vi "query_vectorsearch.vi"(0 "abstract_vector_base in":refnum<class "abstract_vector_base.lvclass">, 5 "collection_name":string, 7 "vector":dbl[](array[numeric]), 9 "limit":u32, 11 "error in (no error)":errorcluster) -> (4 "abstract_vector_base out":refnum<class "abstract_vector_base.lvclass">, 6 "results":T1[](array[typedef]), 15 "error out":errorcluster)   [LabVIEW 2020, in "abstract_vector_base.lvclass"]
uses:
  abstract_vector_base.lvclass
  search result.ctl
  vector.ctl
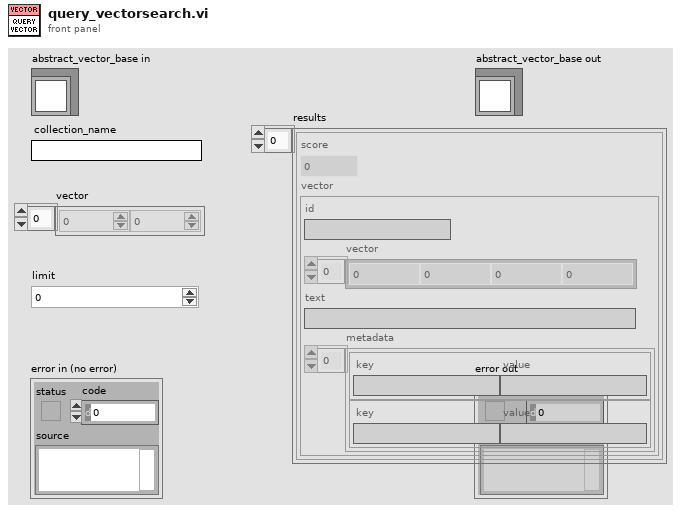
[diagram p1: front panel]
types:
  T1 = typedef "abstract_vector_base.lvclass/search result.ctl" = cluster{"score":dbl, "vector":T2}
  T2 = typedef "abstract_vector_base.lvclass/vector.ctl" = cluster{"id":string, "vector":dbl[], "text":string, "metadata":cluster{"key":string, "value":string}[]}
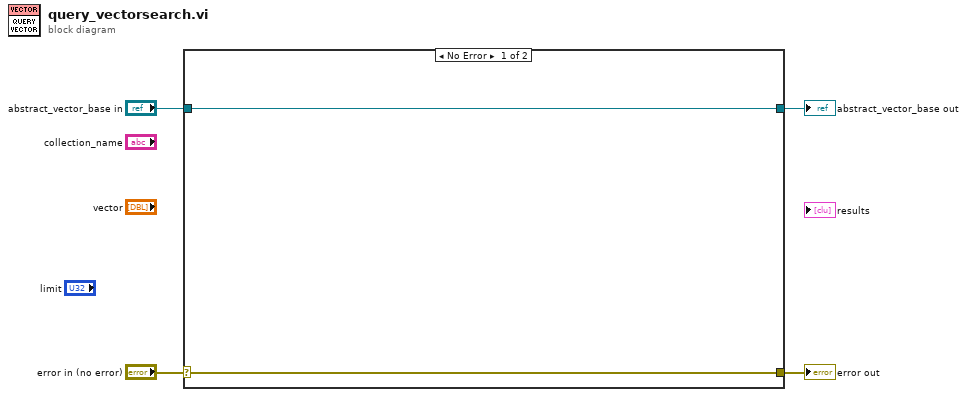
[diagram p0: block diagram]
diagram:
  n1 = case shown="No Error" "error in (no error)" {
    selector: "error in (no error)" -> [w5 w8]
    tunnel: [w5 w8] -> w3
    tunnel: [w6 w7] -> w1
    tunnel: "abstract_vector_base in" -> [w6 w7]
    frame No Error {
    }
    frame Error {
    }
  }
  "error out" <- w3
  "abstract_vector_base out" <- w1
